vi "getApproxValue.vi"(9 "Deflection (mm)":dbl, 11 "data wire":T1 {"x locations" format="%.4g"; "coefficients" format="%.4g"}) -> (2 "Energy (MeV)":dbl)   [LabVIEW 2014]
uses:
  <vilib>/gmath/interp.llb/in_piecewise interp poly control.ctl
  <vilib>/gmath/NI_Gmath.lvlib
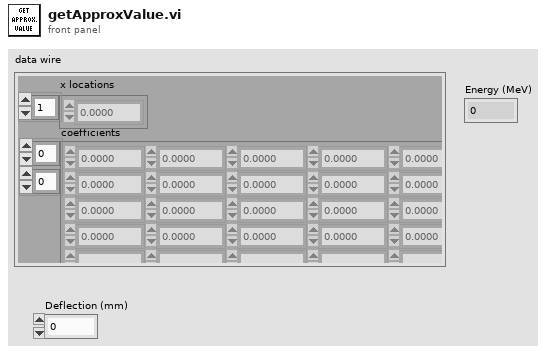
[diagram p1: front panel]
types:
  T1 = typedef "NI_Gmath.lvlib/in_piecewise interp poly control.ctl" = cluster{"x locations":dbl[], "coefficients":dbl[][]}
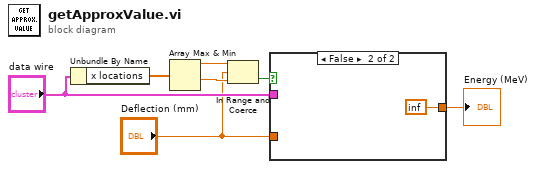
[diagram p0: block diagram]
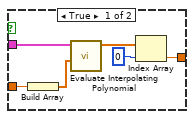
[diagram p2: hidden frame]
diagram:
  n1 = Unbundle By Name("data wire") -> ("x locations"=w4:dbl[])
  n2 = Array Max & Min(array=w4) -> (max value=w6:dbl, min value=w5:dbl)  [unwired: 2 out]
  n3 = In Range and Coerce(upper limit=w6, x="Deflection (mm)", lower limit=w5) -> (In Range?=w3:bool)  [unwired: 1 out]
  n4 = case shown="False" w3 {
    tunnel: [w8 inf] -> w7
    tunnel: "data wire" -> [w13 _]
    tunnel: "Deflection (mm)" -> [w11 _]
    frame True {
      n5 = Build Array(w11) -> (w12:dbl[])
      n6 = call <vilib>:"Evaluate Interpolating Polynomial.vi"("xi"=w12, "piecewise polynomial"=w13) -> ("yi"=w10:dbl[])  [unwired: 8 in, 1 out]
      n7 = Index Array(array=w10, index=0) -> (element=w8:dbl)
    }
    frame False {
    }
  }
  "Energy (MeV)" <- w7
